vi "niDTS WLAN OFDM Tx Test UTIL OFDM ModAcc Settings to WLAN ModAcc Settings.vi"(10 "OFDM ModAcc Measurement Paramaters":T1={"ModAcc Enable"=FALSE, "Header Detection"=enum."MANUAL", "Averages"=0, "CFO Estimation"=enum."PAMBLE", "Amplitude Tracking"=FALSE, "Channel Tracking"=FALSE, "Time Tracking"=FALSE, "Phase Tracking"=enum."NONE", "Clock Offset Est"=TRUE, "Impairments Est"=TRUE}) -> (2 "ModAcc Measurement Paramaters":T2={"ModAcc Enable"=FALSE, "Header Detection"=enum."MANUAL", "Averages"=3, "Amplitude Tracking"=FALSE, "Channel Tracking"=FALSE, "Time Tracking"=TRUE, "Phase Tracking"=enum."NONE", "Clock Offset Est"=FALSE, "Impairments Est"=FALSE, "CFO Estimation"=enum."PAMBLE"})   [LabVIEW 2014, in "niDTS WLAN.lvlib"]
uses:
  niDTS WLAN.lvlib
  Includes/niDTS WLAN INC ModAcc Measurement Parameters.ctl
  Includes/niDTS WLAN OFDM Tx Test INC ModAcc Measurement Parameters.ctl
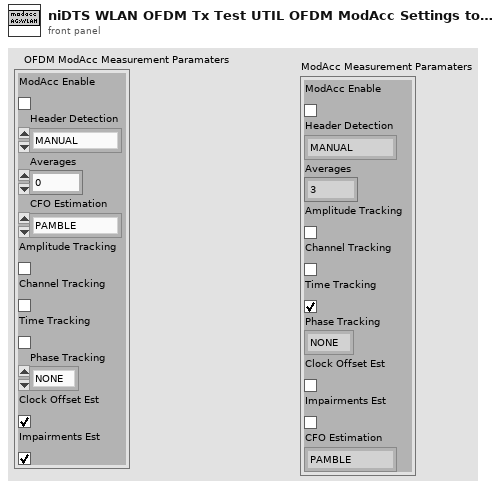
[diagram p1: front panel]
types:
  T1 = typedef "niDTS WLAN.lvlib/niDTS WLAN OFDM Tx Test INC ModAcc Measurement Parameters.ctl" = cluster{"ModAcc Enable":bool, "Header Detection":enum16{"MANUAL", "FIRST", "ALL"}, "Averages":i32, "CFO Estimation":enum16{"PAMBLE", "PDATA"}, "Amplitude Tracking":bool, "Channel Tracking":bool, "Time Tracking":bool, "Phase Tracking":enum16{"NONE", "STANDARD", "CSF", "INSTANT"}, "Clock Offset Est":bool, "Impairments Est":bool}
  T2 = typedef "niDTS WLAN.lvlib/niDTS WLAN INC ModAcc Measurement Parameters.ctl" = cluster{"ModAcc Enable":bool, "Header Detection":enum16{"MANUAL", "FIRST", "ALL"}, "Averages":i32, "Amplitude Tracking":bool, "Channel Tracking":bool, "Time Tracking":bool, "Phase Tracking":enum16{"NONE", "STANDARD", "CSF", "INSTANT"}, "Clock Offset Est":bool, "Impairments Est":bool, "CFO Estimation":enum16{"PAMBLE", "PDATA"}}
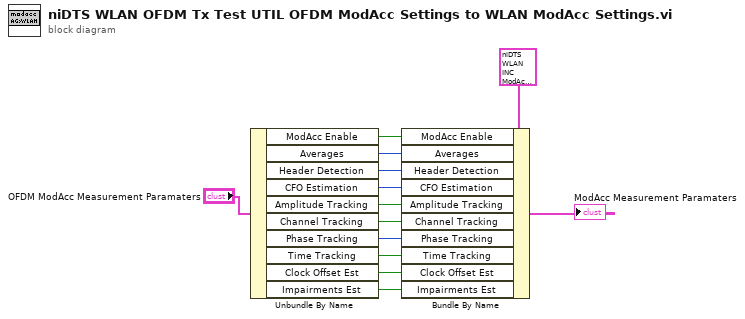
[diagram p0: block diagram]
diagram:
  n1 = Unbundle By Name("OFDM ModAcc Measurement Paramaters") -> ("ModAcc Enable"=w3:bool, "Averages"=w11:i32, "Header Detection"=w10:enum16{"MANUAL", "FIRST", "ALL"}, "CFO Estimation"=w9:enum16{"PAMBLE", "PDATA"}, "Amplitude Tracking"=w8:bool, "Channel Tracking"=w7:bool, "Phase Tracking"=w6:enum16{"NONE", "STANDARD", "CSF", "INSTANT"}, "Time Tracking"=w5:bool, "Clock Offset Est"=w2:bool, "Impairments Est"=w1:bool)
  n2 = Bundle By Name(cluster=T2 {"ModAcc Enable"=FALSE, "Header Detection"=enum."MANUAL", "Averages"=3, "Amplitude Tracking"=FALSE, "Channel Tracking"=FALSE, "Time Tracking"=TRUE, "Phase Tracking"=enum."NONE", "Clock Offset Est"=FALSE, "Impairments Est"=FALSE, "CFO Estimation"=enum."PDATA"} ("ModAcc Measurement Paramaters"), "ModAcc Enable"=w3, "Averages"=w11, "Header Detection"=w10, "CFO Estimation"=w9, "Amplitude Tracking"=w8, "Channel Tracking"=w7, "Phase Tracking"=w6, "Time Tracking"=w5, "Clock Offset Est"=w2, "Impairments Est"=w1) -> (→"ModAcc Measurement Paramaters":T2)
